vi "RS_RF_query.vi"(1 "Parameter":T1(ring), 2 "GPIB address":string="0:19") -> (0 "value":dbl format="%#_24g")   [LabVIEW 2013]
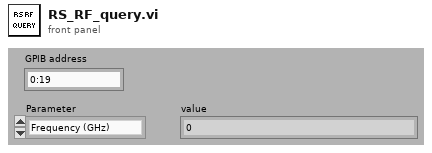
[diagram p1: front panel]
types:
  T1 = enum16{"Frequency (GHz)", "Power (dBm)", "Pulse period (us)", "Pulse width (us)", "Pulse delay (us)", "Pulse modulation?", "Output on?", "Pulse source", "Pulse mode", "Trigger mode", "Ex trigger input slope", "External impedance"}
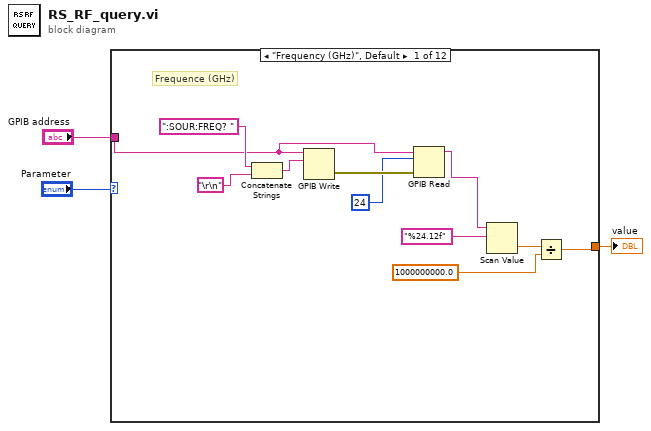
[diagram p0: block diagram]
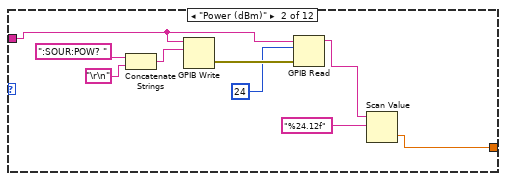
[diagram p2: hidden frame]
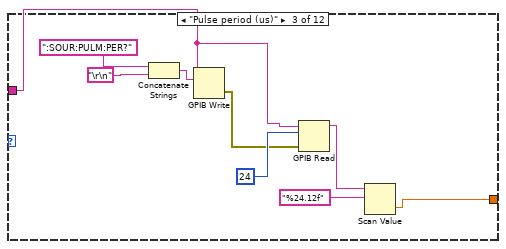
[diagram p3: hidden frame]
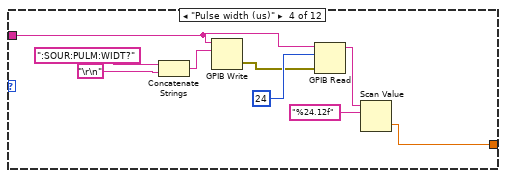
[diagram p4: hidden frame]
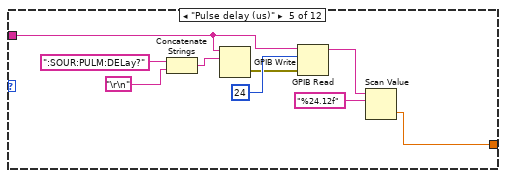
[diagram p5: hidden frame]
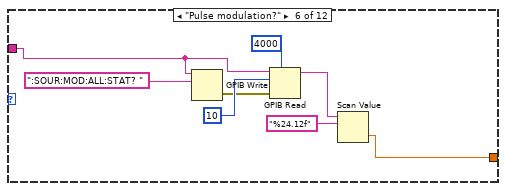
[diagram p6: hidden frame]
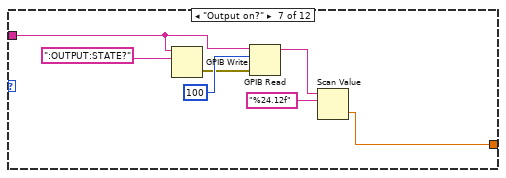
[diagram p7: hidden frame]
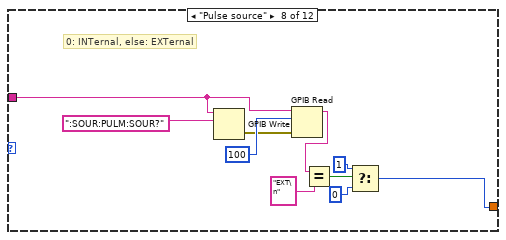
[diagram p8: hidden frame]
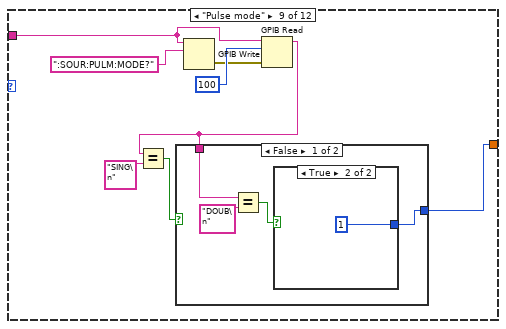
[diagram p9: hidden frame]
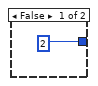
[diagram p10: hidden frame]
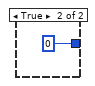
[diagram p11: hidden frame]
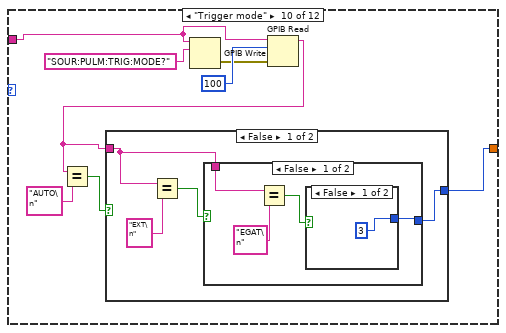
[diagram p12: hidden frame]
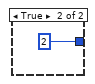
[diagram p13: hidden frame]
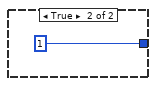
[diagram p14: hidden frame]
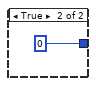
[diagram p15: hidden frame]
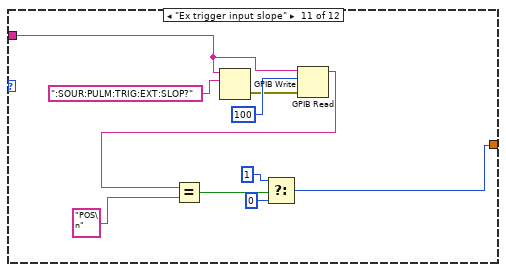
[diagram p16: hidden frame]
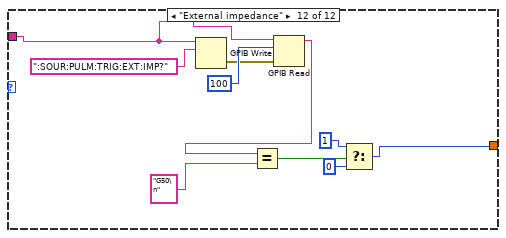
[diagram p17: hidden frame]
diagram:
  n1 = case shown="\"Frequency (GHz)\", Default" "Parameter" {
    tunnel: "GPIB address" -> [w10 w16 w27 w36 w47 w55 w62 w74 w81 w96 w118 w128]
    tunnel: [w5 w15 w24 w33 w43 w53 w60 w66 w77 w91 w111 w121] -> w1
    frame "Frequency (GHz)", Default {
      # "Frequence (GHz)"
      n2 = Concatenate Strings(":SOUR:FREQ? " ("string"), "\r\n") -> (w12:string)
      n3 = GPIB Write(0:w10, 1:w12) -> (6:w11:errorcluster)  [unwired: 3 in, 1 out]
      n4 = GPIB Read(0:w10, 1:24, 3:w11) -> (5:w7:string)  [unwired: 2 in, 2 out]
      n5 = Scan Value(string=w7, format string="%24.12f") -> (value=w6:dbl)  [unwired: 1 in, 1 out]
      n6 = Divide(x=w6, y=1000000000.0) -> (x/y=w5:dbl)
    }
    frame "Power (dBm)" {
      n7 = Concatenate Strings(":SOUR:POW? " ("string"), "\r\n") -> (w17:string)
      n8 = GPIB Write(0:w16, 1:w17) -> (6:w21:errorcluster)  [unwired: 3 in, 1 out]
      n9 = GPIB Read(0:w16, 1:24, 3:w21) -> (5:w18:string)  [unwired: 2 in, 2 out]
      n10 = Scan Value(string=w18, format string="%24.12f") -> (value=w15:dbl)  [unwired: 1 in, 1 out]
    }
    frame "Pulse period (us)" {
      n11 = Concatenate Strings(":SOUR:PULM:PER?" ("string"), "\r\n") -> (w30:string)
      n12 = GPIB Write(0:w27, 1:w30) -> (6:w28:errorcluster)  [unwired: 3 in, 1 out]
      n13 = GPIB Read(0:w27, 1:24, 3:w28) -> (5:w25:string)  [unwired: 2 in, 2 out]
      n14 = Scan Value(string=w25, format string="%24.12f") -> (value=w24:dbl)  [unwired: 1 in, 1 out]
    }
    frame "Pulse width (us)" {
      n15 = Concatenate Strings(":SOUR:PULM:WIDT?" ("string"), "\r\n") -> (w39:string)
      n16 = GPIB Write(0:w36, 1:w39) -> (6:w37:errorcluster)  [unwired: 3 in, 1 out]
      n17 = GPIB Read(0:w36, 1:24, 3:w37) -> (5:w34:string)  [unwired: 2 in, 2 out]
      n18 = Scan Value(string=w34, format string="%24.12f") -> (value=w33:dbl)  [unwired: 1 in, 1 out]
    }
    frame "Pulse delay (us)" {
      n19 = Concatenate Strings(":SOUR:PULM:DELay?" ("string"), "\r\n") -> (w48:string)
      n20 = GPIB Write(0:w47, 1:w48) -> (6:w42:errorcluster)  [unwired: 3 in, 1 out]
      n21 = GPIB Read(0:w47, 1:24, 3:w42) -> (5:w44:string)  [unwired: 2 in, 2 out]
      n22 = Scan Value(string=w44, format string="%24.12f") -> (value=w43:dbl)  [unwired: 1 in, 1 out]
    }
    frame "Pulse modulation?" {
      n23 = GPIB Write(0:w55, 1:":SOUR:MOD:ALL:STAT? " ("string")) -> (6:w51:errorcluster)  [unwired: 3 in, 1 out]
      n24 = GPIB Read(0:w55, 1:10, 3:w51, 4:4000) -> (5:w56:string)  [unwired: 1 in, 2 out]
      n25 = Scan Value(string=w56, format string="%24.12f") -> (value=w53:dbl)  [unwired: 1 in, 1 out]
    }
    frame "Output on?" {
      n26 = GPIB Write(0:w62, 1:":OUTPUT:STATE?") -> (6:w59:errorcluster)  [unwired: 3 in, 1 out]
      n27 = GPIB Read(0:w62, 1:100, 3:w59) -> (5:w63:string)  [unwired: 2 in, 2 out]
      n28 = Scan Value(string=w63, format string="%24.12f") -> (value=w60:dbl)  [unwired: 1 in, 1 out]
    }
    frame "Pulse source" {
      # "0: INTernal, else: EXTernal"
      n29 = GPIB Write(0:w74, 1:":SOUR:PULM:SOUR?") -> (6:w72:errorcluster)  [unwired: 3 in, 1 out]
      n30 = GPIB Read(0:w74, 1:100, 3:w72) -> (5:w70:string)  [unwired: 2 in, 2 out]
      n31 = Equal?(x=w70, y="EXT\n") -> (x = y?=w71:bool)
      n32 = Select(t=1, s=w71, f=0) -> (s? t:f=w66:i32)
    }
    frame "Pulse mode" {
      n33 = GPIB Write(0:w81, 1:":SOUR:PULM:MODE?") -> (6:w80:errorcluster)  [unwired: 3 in, 1 out]
      n34 = GPIB Read(0:w81, 1:100, 3:w80) -> (5:w76:string)  [unwired: 2 in, 2 out]
      n35 = Equal?(x=w76, y="SING\n") -> (x = y?=w78:bool)
      n36 = case shown="False" w78 {
        tunnel: [w84 0] -> w77
        tunnel: w76 -> [w86 _]
        frame False {
          n37 = Equal?(x=w86, y="DOUB\n") -> (x = y?=w85:bool)
          n38 = case shown="True" w85 {
            tunnel: [2 1] -> w84
            frame False {
            }
            frame True {
            }
          }
        }
        frame True {
        }
      }
    }
    frame "Trigger mode" {
      n39 = GPIB Write(0:w96, 1:"SOUR:PULM:TRIG:MODE?") -> (6:w95:errorcluster)  [unwired: 3 in, 1 out]
      n40 = GPIB Read(0:w96, 1:100, 3:w95) -> (5:w92:string)  [unwired: 2 in, 2 out]
      n41 = Equal?(x=w92, y="AUTO\n") -> (x = y?=w93:bool)
      n42 = case shown="False" w93 {
        tunnel: w92 -> [w99 _]
        tunnel: [w100 0] -> w91
        frame False {
          n43 = Equal?(x=w99, y="EXT\n") -> (x = y?=w101:bool)
          n44 = case shown="False" w101 {
            tunnel: [w103 1] -> w100
            tunnel: w99 -> [w105 _]
            frame False {
              n45 = Equal?(x=w105, y="EGAT\n") -> (x = y?=w104:bool)
              n46 = case shown="False" w104 {
                tunnel: [3 2] -> w103
                frame False {
                }
                frame True {
                }
              }
            }
            frame True {
            }
          }
        }
        frame True {
        }
      }
    }
    frame "Ex trigger input slope" {
      n47 = GPIB Write(0:w118, 1:":SOUR:PULM:TRIG:EXT:SLOP?") -> (6:w117:errorcluster)  [unwired: 3 in, 1 out]
      n48 = GPIB Read(0:w118, 1:100, 3:w117) -> (5:w116:string)  [unwired: 2 in, 2 out]
      n49 = Equal?(x=w116, y="POS\n") -> (x = y?=w114:bool)
      n50 = Select(t=1, s=w114, f=0) -> (s? t:f=w111:i32)
    }
    frame "External impedance" {
      n51 = GPIB Write(0:w128, 1:":SOUR:PULM:TRIG:EXT:IMP?") -> (6:w127:errorcluster)  [unwired: 3 in, 1 out]
      n52 = GPIB Read(0:w128, 1:100, 3:w127) -> (5:w122:string)  [unwired: 2 in, 2 out]
      n53 = Equal?(x=w122, y="G50\n") -> (x = y?=w125:bool)
      n54 = Select(t=1, s=w125, f=0) -> (s? t:f=w121:i32)
    }
  }
  "value" <- w1
